vi "Write Install after build.vi"(8 "error in (no error)":errorcluster, 10 "Install after build":bool, 11 "VIPB Build in":refnum<class "VIPB Build.lvclass">) -> (0 "error out":errorcluster, 3 "VIPB Build out":refnum<class "VIPB Build.lvclass">)   [LabVIEW 2014, in "VIPB Build.lvclass"]
uses:
  VIPB Build.lvclass
  VIPB Build.lvclass/VIPB Build.ctl
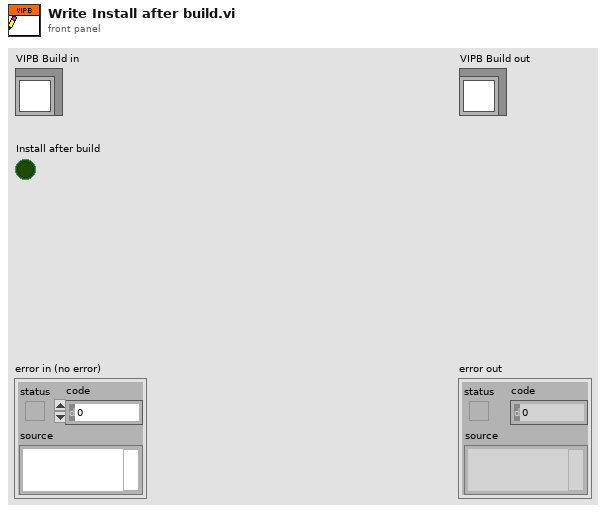
[diagram p1: front panel]
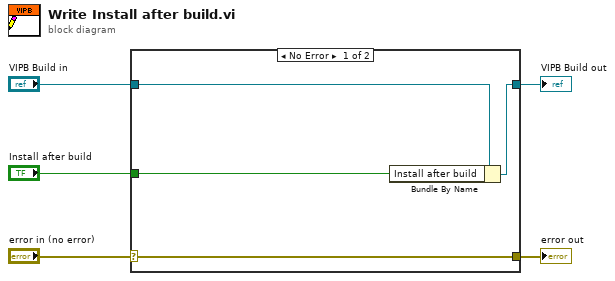
[diagram p0: block diagram]
diagram:
  n1 = case shown="No Error" "error in (no error)" {
    selector: "error in (no error)" -> [w9 w10]
    tunnel: [w9 w10] -> w4
    tunnel: [w7 w11] -> w2
    tunnel: "VIPB Build in" -> [w8 w11]
    tunnel: "Install after build" -> [w6 _]
    frame No Error {
      n2 = Bundle By Name(cluster=w8, "Install after build"=w6) -> (w7:refnum<class "VIPB Build.lvclass">)
    }
    frame Error {
    }
  }
  "error out" <- w4
  "VIPB Build out" <- w2
